vi "ziModGetSweeperData.vi"(8 "Error In":errorcluster, 10 "ModResults":T4, 11 "ModHandle In":T7 {"ModHandle" format="0x%08x"; "Conn" format="0x%08x"}) -> (0 "Error Out":errorcluster, 1 "SweeperImpedanceWaveArray":T2[](array[typedef]) {"bandwidthMode" format="%f"; "flags" format="%f"; "sampleFormat" format="%f"; "sweepMode" format="%f"; "sampleCount" format="%f"; "timestamp" format="%f"}, 2 "SweeperDemodWaveArray":T3[](array[typedef]) {"bandwidthMode" format="%f"; "flags" format="%f"; "sampleFormat" format="%f"; "sweepMode" format="%f"; "sampleCount" format="%f"; "timestamp" format="%f"}, 3 "ModHandle Out":T7 {"ModHandle" format="0x%08x"; "Conn" format="0x%08x"}, 4 "SweeperDoubleWaveArray":T1[](array[typedef]) {"bandwidthMode" format="%f"; "flags" format="%f"; "sampleFormat" format="%f"; "sweepMode" format="%f"; "sampleCount" format="%f"; "timestamp" format="%f"})   [LabVIEW 2018, in "Zurich Instruments LabOne.lvlib"]
doc: "Use this vi to get SweeperData from a ModResult returned from ziModGetNextNode.vi is used. It return an array of SweeperData."
uses:
  Zurich Instruments LabOne.lvlib
  ziTypeModHandle.ctl
  ziTypeModResults.ctl
  Data/ziTypePollType.ctl
  ziTypeModGenericHeader.ctl
  ziTypeModSweeperDemodWave.ctl
  ziTypeModSweeperImpedanceWave.ctl
  ziTypeModSweeperDoubleWave.ctl
  ziLV32.dll
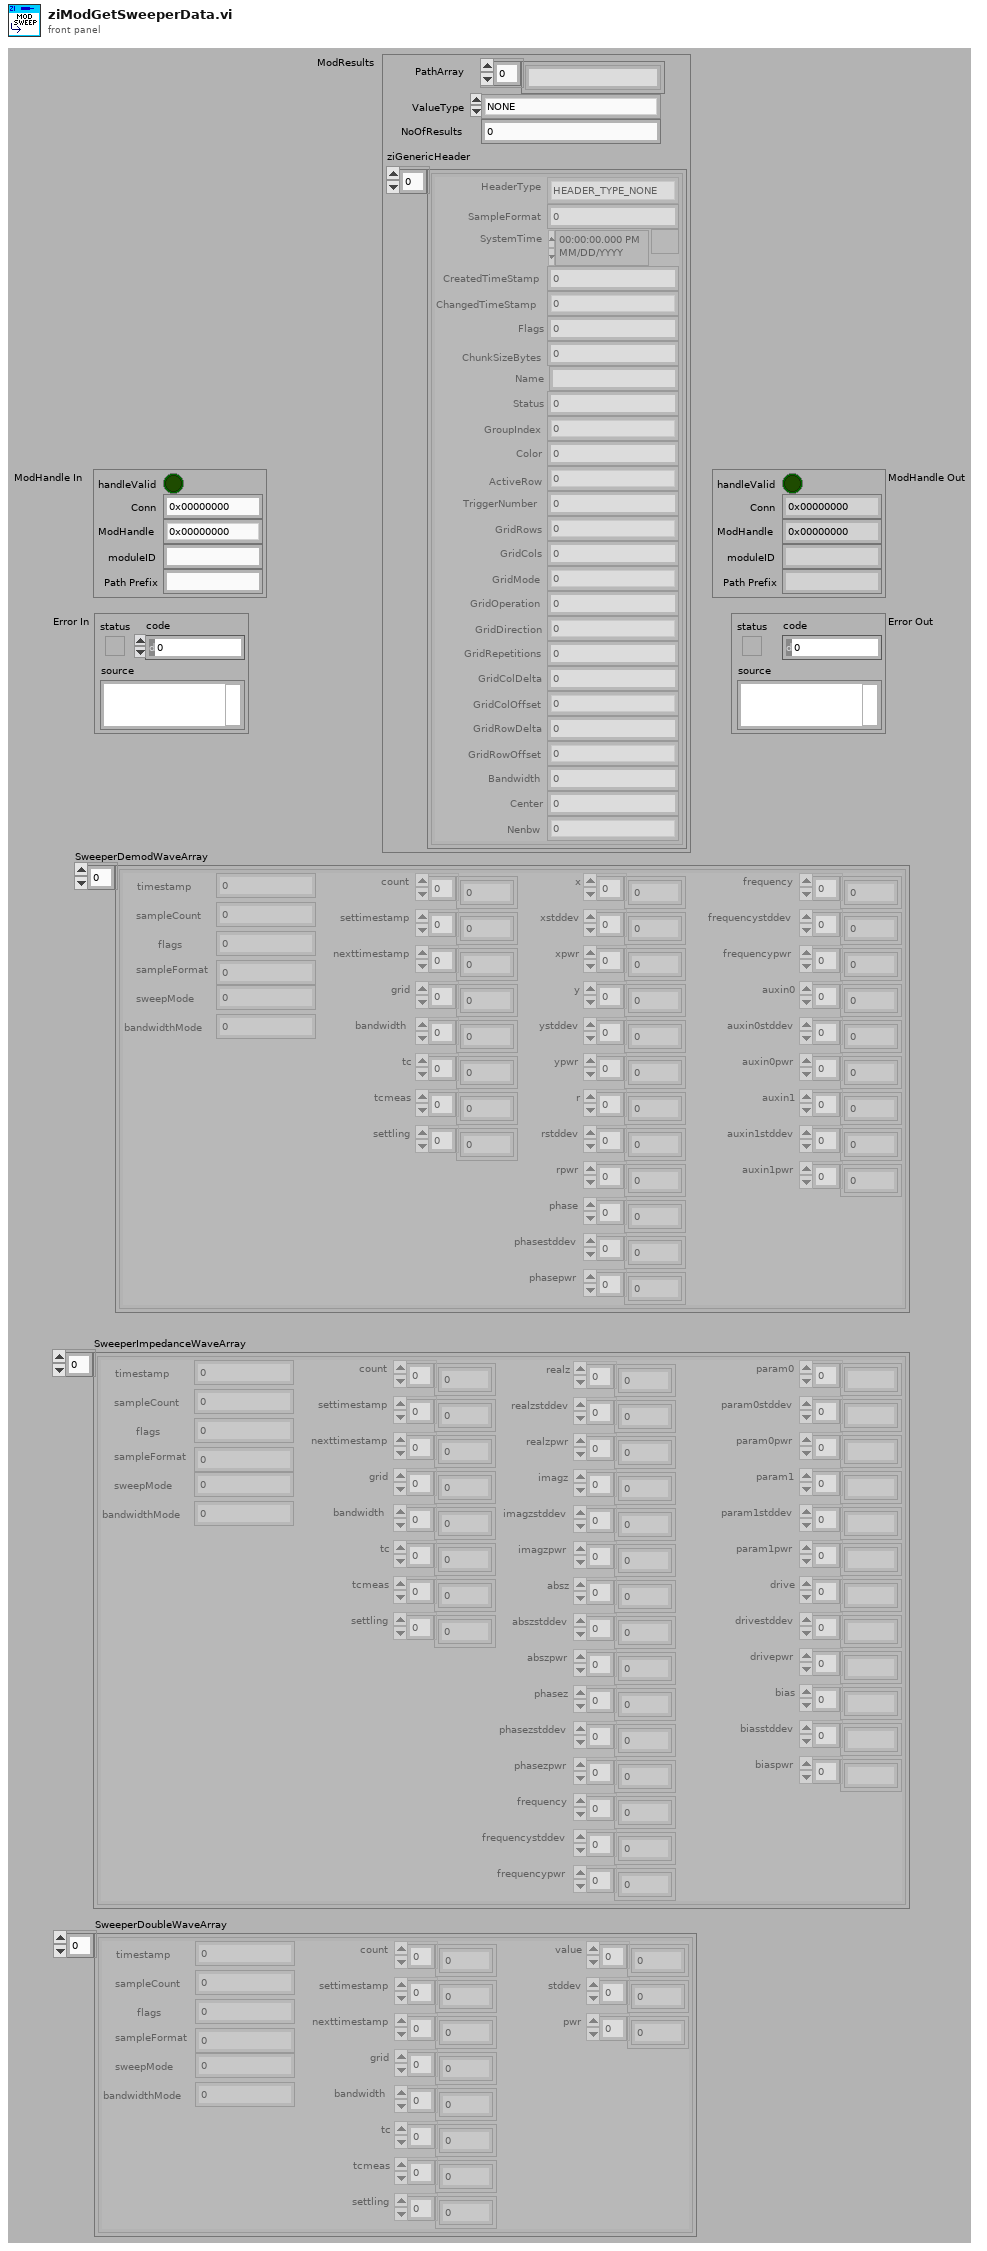
[diagram p1: front panel]
types:
  T1 = typedef "Zurich Instruments LabOne.lvlib/ziTypeModSweeperDoubleWave.ctl" = cluster{"timestamp":u64, "sampleCount":u64, "flags":u8, "sampleFormat":u8, "sweepMode":u8, "bandwidthMode":u8, "count":u64[], "settimestamp":u64[], "nexttimestamp":u64[], "grid":dbl[], "bandwidth":dbl[], "tc":dbl[], "tcmeas":dbl[], "settling":dbl[], "value":dbl[], "stddev":dbl[], "pwr":dbl[]}
  T2 = typedef "Zurich Instruments LabOne.lvlib/ziTypeModSweeperImpedanceWave.ctl" = cluster{"timestamp":u64, "sampleCount":u64, "flags":u8, "sampleFormat":u8, "sweepMode":u8, "bandwidthMode":u8, "count":u64[], "settimestamp":u64[], "nexttimestamp":u64[], "grid":dbl[], "bandwidth":dbl[], "tc":dbl[], "tcmeas":dbl[], "settling":dbl[], "realz":dbl[], "realzstddev":dbl[], "realzpwr":dbl[], "imagz":dbl[], "imagzstddev":dbl[], "imagzpwr":dbl[], "absz":dbl[], "abszstddev":dbl[], "abszpwr":dbl[], "phasez":dbl[], "phasezstddev":dbl[], "phasezpwr":dbl[], "frequency":dbl[], "frequencystddev":dbl[], "frequencypwr":dbl[], "param0":dbl[], "param0stddev":dbl[], "param0pwr":dbl[], "param1":dbl[], "param1stddev":dbl[], "param1pwr":dbl[], "drive":dbl[], "drivestddev":dbl[], "drivepwr":dbl[], "bias":dbl[], "biasstddev":dbl[], "biaspwr":dbl[]}
  T3 = typedef "Zurich Instruments LabOne.lvlib/ziTypeModSweeperDemodWave.ctl" = cluster{"timestamp":u64, "sampleCount":u64, "flags":u8, "sampleFormat":u8, "sweepMode":u8, "bandwidthMode":u8, "count":u64[], "settimestamp":u64[], "nexttimestamp":u64[], "grid":dbl[], "bandwidth":dbl[], "tc":dbl[], "tcmeas":dbl[], "settling":dbl[], "x":dbl[], "xstddev":dbl[], "xpwr":dbl[], "y":dbl[], "ystddev":dbl[], "ypwr":dbl[], "r":dbl[], "rstddev":dbl[], "rpwr":dbl[], "phase":dbl[], "phasestddev":dbl[], "phasepwr":dbl[], "frequency":dbl[], "frequencystddev":dbl[], "frequencypwr":dbl[], "auxin0":dbl[], "auxin0stddev":dbl[], "auxin0pwr":dbl[], "auxin1":dbl[], "auxin1stddev":dbl[], "auxin1pwr":dbl[]}
  T4 = typedef "Zurich Instruments LabOne.lvlib/ziTypeModResults.ctl" = cluster{"PathArray":string[], "ValueType":T5, "NoOfResults":u64, "ziGenericHeader":T6[]}
  T5 = typedef "Zurich Instruments LabOne.lvlib/ziTypePollType.ctl" = enum16{"NONE", "DOUBLE_DATA", "INTEGER_DATA", "DEMOD_SAMPLE", "SCOPE_WAVE_HF2", "AUXIN_SAMPLE", "DIO_SAMPLE", "BYTE_ARRAY", "PWA_WAVE", "9", "10", "11", "12", "13", "14", "15", "TREE_CHANGE_DEPRI", "17", "ERROR", "19", "20", "21", "22", "23", "24", "25", "26", "27", "28", "29", "30", "31", "DOUBLE_DATA_TS", "INTEGER_DATA_TS", "34", "SCOPE_WAVE", "SCOPE_WAVE_EX", "37", "BYTE_ARRAY_TS", "39", "40", "41", "42", "43", "44", "45", "CNT_DATA", "47", "TREE_CHANGE", "49", "50", "51", "52", "53", "54", "55", "56", "57", "58", "59", "60", "61", "62", "63", "SWEEPER_DATA", "SPECTRUM_DATA", "ADVISOR_DATA", "VECTOR_DATA", "IMP_DATA"}
  T6 = typedef "Zurich Instruments LabOne.lvlib/ziTypeModGenericHeader.ctl" = cluster{"HeaderType":enum8{"HEADER_TYPE_NONE", "HEADER_TYPE_SWTRIGGER", "HEADER_TYPE_SWEEPER"}, "SampleFormat":u8, "SystemTime":timestamp, "CreatedTimeStamp":u64, "ChangedTimeStamp":u64, "Flags":u32, "ChunkSizeBytes":u64, "Name":string, "Status":u32, "GroupIndex":u32, "Color":u32, "ActiveRow":u32, "TriggerNumber":u64, "GridRows":u32, "GridCols":u32, "GridMode":u32, "GridOperation":u32, "GridDirection":u32, "GridRepetitions":u32, "GridColDelta":dbl, "GridColOffset":dbl, "GridRowDelta":dbl, "GridRowOffset":dbl, "Bandwidth":dbl, "Center":dbl, "Nenbw":dbl}
  T7 = typedef "Zurich Instruments LabOne.lvlib/ziTypeModHandle.ctl" = cluster{"handleValid":bool, "Conn":u64, "ModHandle":u64, "moduleID":string, "Path Prefix":string}
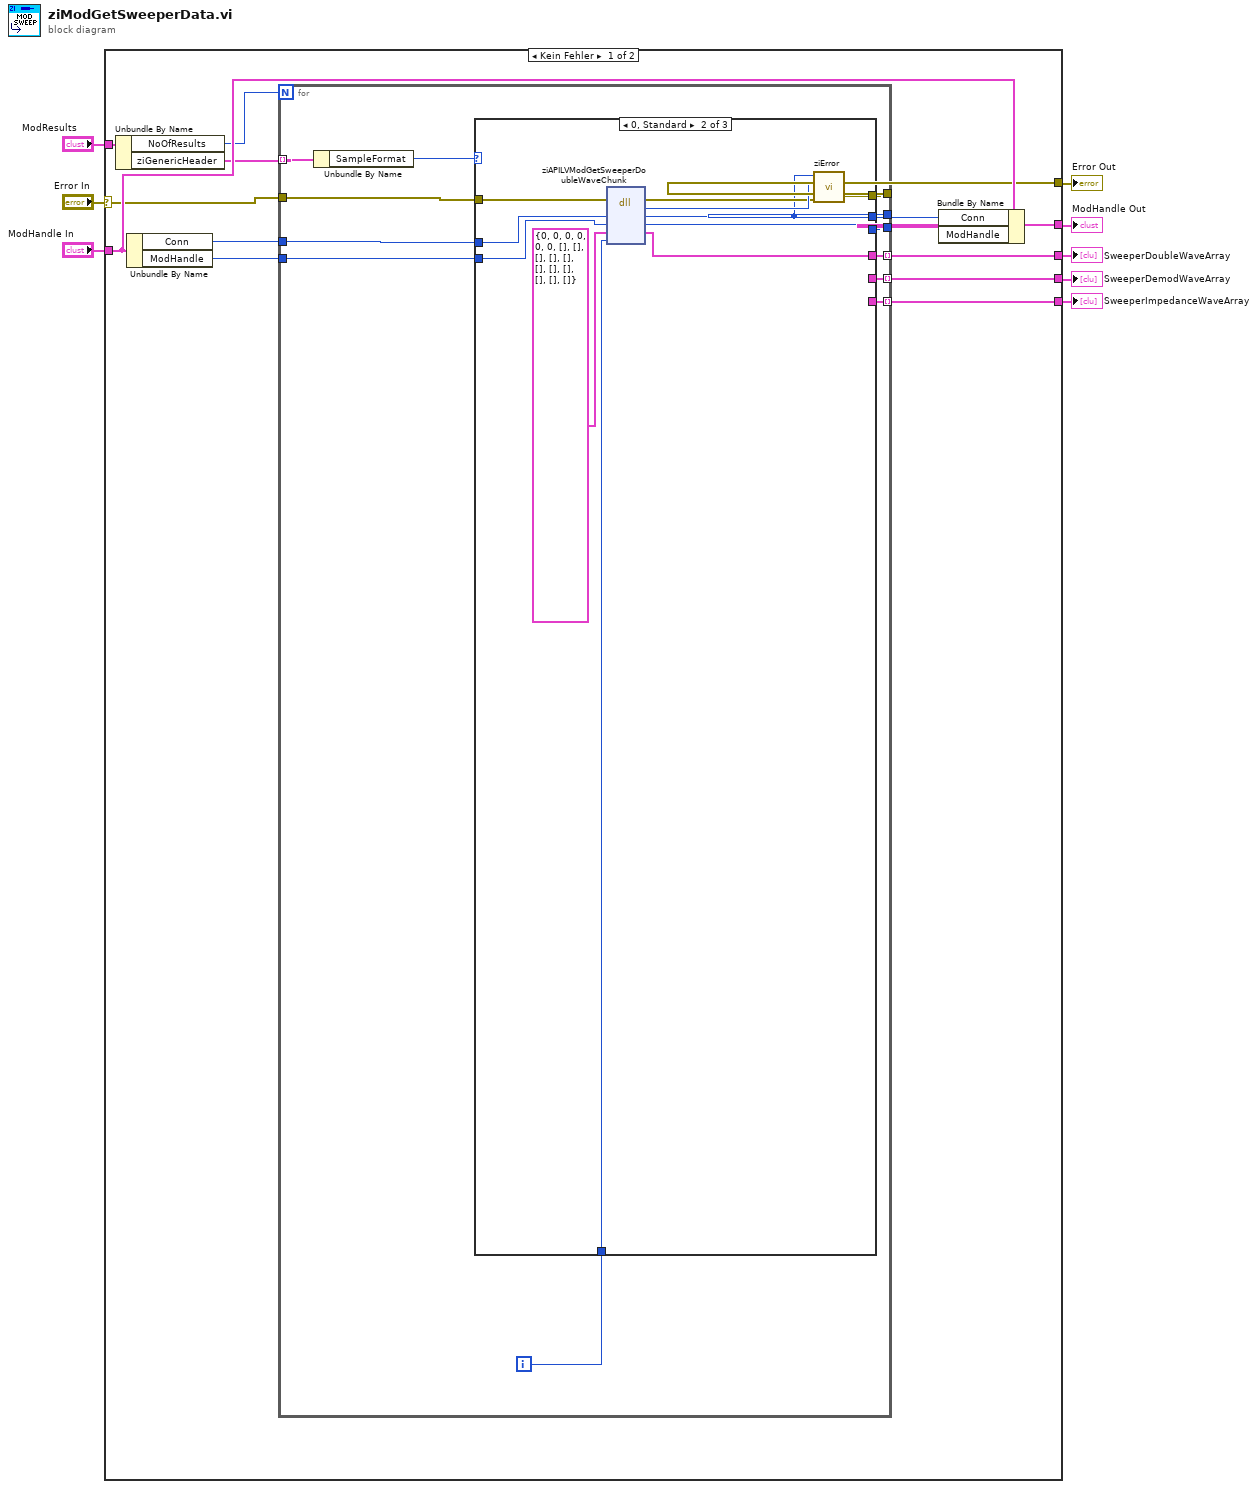
[diagram p0: block diagram]
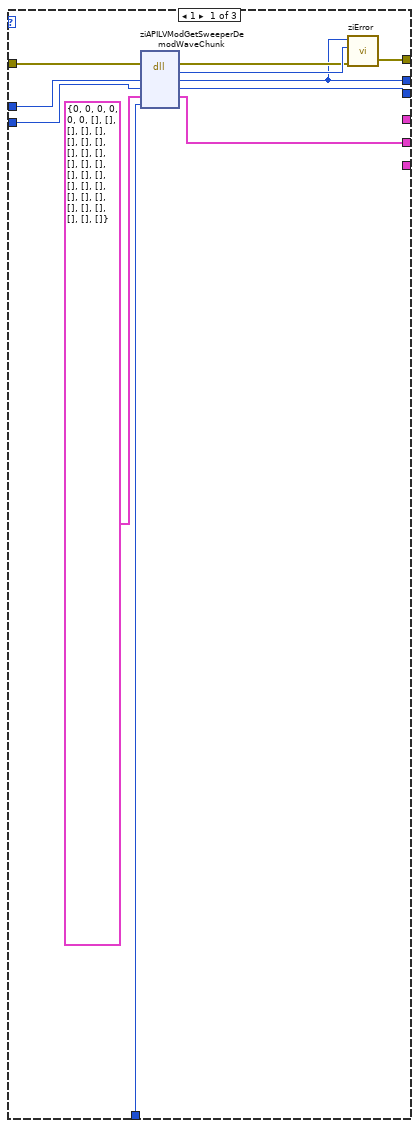
[diagram p2: hidden frame]
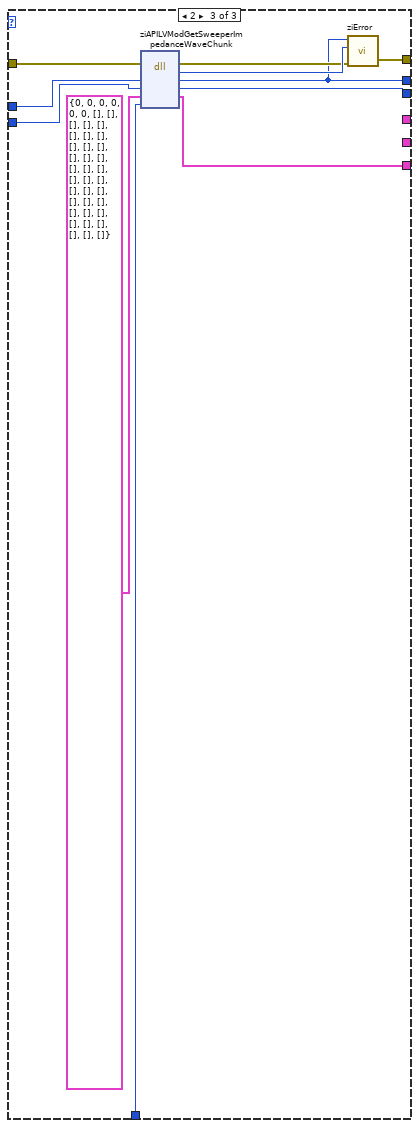
[diagram p3: hidden frame]
diagram:
  n1 = case shown="Kein Fehler" "Error In" {
    selector: "Error In" -> [w13 w68]
    tunnel: [w14 w68] -> w4
    tunnel: [w21 w69] -> w7
    tunnel: "ModHandle In" -> [w22 w69]
    tunnel: "ModResults" -> [w18 _]
    tunnel: [w12 _] -> w3
    tunnel: [w10 _] -> w2
    tunnel: [w9 _] -> w1
    frame No Error {
      n2 = Unbundle By Name(w18) -> ("NoOfResults"=w17:u64, "ziGenericHeader"=w11:T6[])
      n3 = Unbundle By Name(w22) -> ("Conn"=w20:u64, "ModHandle"=w19:u64)
      n4 = for {
        N: w17 -> [_]
        tunnel: [w27] -> w16
        tunnel: [w34] -> w15
        tunnel: w20 -> [w33]
        tunnel: w19 -> [w32]
        tunnel: [w30] -> w14
        tunnel: w13 -> [w29]
        tunnel: [w28] -> w12 mode=indexing
        tunnel: w11 -> [w26] mode=indexing
        tunnel: [w24] -> w10 mode=indexing
        tunnel: [w23] -> w9 mode=indexing
        i -> [w31]
        n5 = Unbundle By Name(w26) -> ("SampleFormat"=w25:u8)
        n6 = case shown="0, Standard" w25 {
          tunnel: [w45 w56 w67] -> w34
          tunnel: w33 -> [w44 w55 w66]
          tunnel: w32 -> [w43 w54 w65]
          tunnel: w31 -> [w42 w53 w64]
          tunnel: [w40 w51 w62] -> w30
          tunnel: w29 -> [w37 w48 w59]
          tunnel: [w36 _ _] -> w28
          tunnel: [w35 w47 w58] -> w27
          tunnel: [_ _ w57] -> w24
          tunnel: [_ w46 _] -> w23
          frame 1 {
            n7 = dll-call lib="ziLV*.*" fn="ziAPILVModGetSweeperDemodWaveChunk"(error in=w37, "Conn"=w44, "ModHandle"=w43, "SweeperWave"=T3 {"timestamp"=0, "sampleCount"=0, "flags"=0, "sampleFormat"=0, "sweepMode"=0, "bandwidthMode"=0, "count"=[], "settimestamp"=[], "nexttimestamp"=[], "grid"=[], "bandwidth"=[], "tc"=[], "tcmeas"=[], "settling"=[], "x"=[], "xstddev"=[], "xpwr"=[], "y"=[], "ystddev"=[], "ypwr"=[], "r"=[], "rstddev"=[], "rpwr"=[], "phase"=[], "phasestddev"=[], "phasepwr"=[], "frequency"=[], "frequencystddev"=[], "frequencypwr"=[], "auxin0"=[], "auxin0stddev"=[], "auxin0pwr"=[], "auxin1"=[], "auxin1stddev"=[], "auxin1pwr"=[]} ("ziModSweeperWave Out 2"), "chunk_idx"=w42) -> (error out=w38:errorcluster, "return type"=w39:u32, "Conn"=w35:u64, "ModHandle"=w45:u64, "SweeperWave"=w36:T3)  [unwired: 3 in, 1 out]
            n8 = call "ziError.vi"("Conn"=w35, "ziErrorCode"=w39, "Error In"=w38) -> ("Error Out"=w40:errorcluster)  [unwired: 2 in, 1 out]
          }
          frame 0, Default {
            n9 = dll-call lib="ziLV*.*" fn="ziAPILVModGetSweeperDoubleWaveChunk"(error in=w48, "Conn"=w55, "ModHandle"=w54, "SweeperWave"=T1 {"timestamp"=0, "sampleCount"=0, "flags"=0, "sampleFormat"=0, "sweepMode"=0, "bandwidthMode"=0, "count"=[], "settimestamp"=[], "nexttimestamp"=[], "grid"=[], "bandwidth"=[], "tc"=[], "tcmeas"=[], "settling"=[], "value"=[], "stddev"=[], "pwr"=[]} ("ziModSweeperWave Out 2"), "chunk_idx"=w53) -> (error out=w49:errorcluster, "return type"=w50:u32, "Conn"=w47:u64, "ModHandle"=w56:u64, "SweeperWave"=w46:T1)  [unwired: 3 in, 1 out]
            n10 = call "ziError.vi"("Conn"=w47, "ziErrorCode"=w50, "Error In"=w49) -> ("Error Out"=w51:errorcluster)  [unwired: 2 in, 1 out]
          }
          frame 2 {
            n11 = dll-call lib="ziLV*.*" fn="ziAPILVModGetSweeperImpedanceWaveChunk"(error in=w59, "Conn"=w66, "ModHandle"=w65, "SweeperWave"=T2 {"timestamp"=0, "sampleCount"=0, "flags"=0, "sampleFormat"=0, "sweepMode"=0, "bandwidthMode"=0, "count"=[], "settimestamp"=[], "nexttimestamp"=[], "grid"=[], "bandwidth"=[], "tc"=[], "tcmeas"=[], "settling"=[], "realz"=[], "realzstddev"=[], "realzpwr"=[], "imagz"=[], "imagzstddev"=[], "imagzpwr"=[], "absz"=[], "abszstddev"=[], "abszpwr"=[], "phasez"=[], "phasezstddev"=[], "phasezpwr"=[], "frequency"=[], "frequencystddev"=[], "frequencypwr"=[], "param0"=[], "param0stddev"=[], "param0pwr"=[], "param1"=[], "param1stddev"=[], "param1pwr"=[], "drive"=[], "drivestddev"=[], "drivepwr"=[], "bias"=[], "biasstddev"=[], "biaspwr"=[]} ("ziModSweeperWave Out 2"), "chunk_idx"=w64) -> (error out=w60:errorcluster, "return type"=w61:u32, "Conn"=w58:u64, "ModHandle"=w67:u64, "SweeperWave"=w57:T2)  [unwired: 3 in, 1 out]
            n12 = call "ziError.vi"("Conn"=w58, "ziErrorCode"=w61, "Error In"=w60) -> ("Error Out"=w62:errorcluster)  [unwired: 2 in, 1 out]
          }
        }
      }
      n13 = Bundle By Name(cluster=w22, "Conn"=w16, "ModHandle"=w15) -> (w21:T7)
    }
    frame Error {
    }
  }
  "Error Out" <- w4
  "ModHandle Out" <- w7
  "SweeperDemodWaveArray" <- w3
  "SweeperImpedanceWaveArray" <- w2
  "SweeperDoubleWaveArray" <- w1
